vi "Agilent_33220A_FuncGen_TCP.vi"() -> ()   [LabVIEW 2019, in "Models of External Instruments.lvlib"]
uses:
  Models of External Instruments.lvlib
panel:
  out "remote address":string
  out "remote port":u16
  out "data out 2":string
  in  "data in":string
  out "bytes written":i32
  out "data out":string
  # "Output Configuration Commands\n\nOUTP ON\nOUTP OFF \n\nOUTP? --> 1 ON, 0 OFF\n\nOUTP:LOAD? -->yük empedansı\nOUTP:LOAD?  MAX--> maks yük empedansı\nOUTP:LOAD?  MIN--> min yük empedansı\n\nOUTP:POL? --> Normal or Inverted\nOUTP:POL INV -->Inverted waveform\nOUTP:POL?\n\nOUTP:POL NORM-->Normal Waveform\nOUTP:POL?\n\nOUTP:SYNC ON  -->Sync konnectörünü aktif eder\nOUTP:SYNC OFF -->Sync konnectörünü deaktif eder\nOUTP:SYNC? --> Sync konnectörünün durumu 1-ON, 0-OFF\n\nVOLT:UNIT? --> Voltaj biriminin durumu\nVOLT:UNIT VRMS -->birim Vrms\nVOLT:UNIT VPP -->birim Vpp\nVOLT:UNIT DBM -->birim dBm"
  # "Pulse Configuration Commands\n\nPULS:PER 5  --> saniye cinsinden darbe periydunun ayarı\nPULS:PER MIN --> Minimumu 200ns olarak ayarlar\nPULS:PER MAX --> Maxı 2000s olarak ayarlar\nPULS:PER? -*->pulse periyot durumu\n\nFUNC:PULSE:HOLD WID --> pulse genişliği şeklinde ayarla\nFUNC:PULSE:HOLD DCYC --> pulse duty cycle şeklinde ayarla\nFUNC:PULSE:HOLD -->Pulse ayar durumu\n\nFUNC:PULS:WIDT 5-->Pulse genişliği saniye cinsinden ayarla\nFUNC:PULS:WIDT MAX --> Pulse genişliğini max 1999.99 s olarak ayarla\nFUNC:PULS:WIDT MIN --> Pulse genişliğini min 20ns olarak ayarla\nFUNC:PULS:WIDT? --> Pulse genişliğinin durumu\n\nFUNC:PULS:DCYC 50-->Pulse duty cycle'ını oran cinsinden ayarla\nFUNC:PULS:DCYC MAX -->Pulse duty cycle'ını max 100% olarak ayarla\nFUNC:PULS:DCYC MIN --> Pulse duty cycle'ını  min 0% olarak ayarla\nFUNC:PULS:DCYC? -->  Pulse duty cycle'ının durumu\n\nFUNC:PULS:TRAN 50 --> düşen ve yükselen kenar için edge time'ı oran olarak ayarla\n                                             edge time from 5 ns to 100 ns\nFUNC:PULS:TRAN MAX --> edge time 100ns\nFUNC:PULS:TRAN MIN --> edge time 5ns\nFUNC:PULS:TRAN? -->edge time durumu"
  # "APPLy Command\n\nAPPL:SIN 5 KHZ, 3.0 VPP, -2.5 V\nAPPL?\n\nAPPL:SIN 5.0E+3, 3.0 VRMS, -2.5\nAPPL?\n\nAPPL:SQU 5.0E+3, 3.0, -2.5\nAPPL?"
  # "APPLy\n:SINusoid [<frequency> [,<amplitude> [,<offset>] ]]\n:SQUare [<frequency> [,<amplitude> [,<offset>] ]]\n:RAMP [<frequency> [,<amplitude> [,<offset>] ]]\n:PULSe [<frequency> [,<amplitude> [,<offset>] ]]\n:NOISe [<frequency|DEF>1 [,<amplitude> [,<offset>] ]]\n:DC [<frequency|DEF>1 [,<amplitude>|DEF>1 [,<offset>] ]]\n:USER [<frequency> [,<amplitude> [,<offset>] ]]\nAPPLy?"
  # "Low-Level Commands\n\nFUNC SIN --> Select sine wave function\nFREQ 5000 -->Set frequency to 5 kHz\nVOLT 3.0 --> Set amplitude to 3 Vpp\nVOLT:OFFS -2.5 --> Set offset to -2.5 Vdc\nAPPL?"
  # "*IDN? --> cihaz bilgileri: Agilent Technologies,33220A,<serial number>,f.ff-b.bb-aa-p\n                                            f.ff = Firmware revision number\n                                            b.bb = Boot kernel revision number\n                                            aa = ASIC revision number\n                                            p = Printed circuit board revision number\nSYSTem:VERSion? --> sistem verisyonu\n\nSYST:ERR? --> Hataları oku\n\nDISP ON--> ekranı aç\nDISP OFF--> ekranı kapat\nDISP? --> ekran durumu"
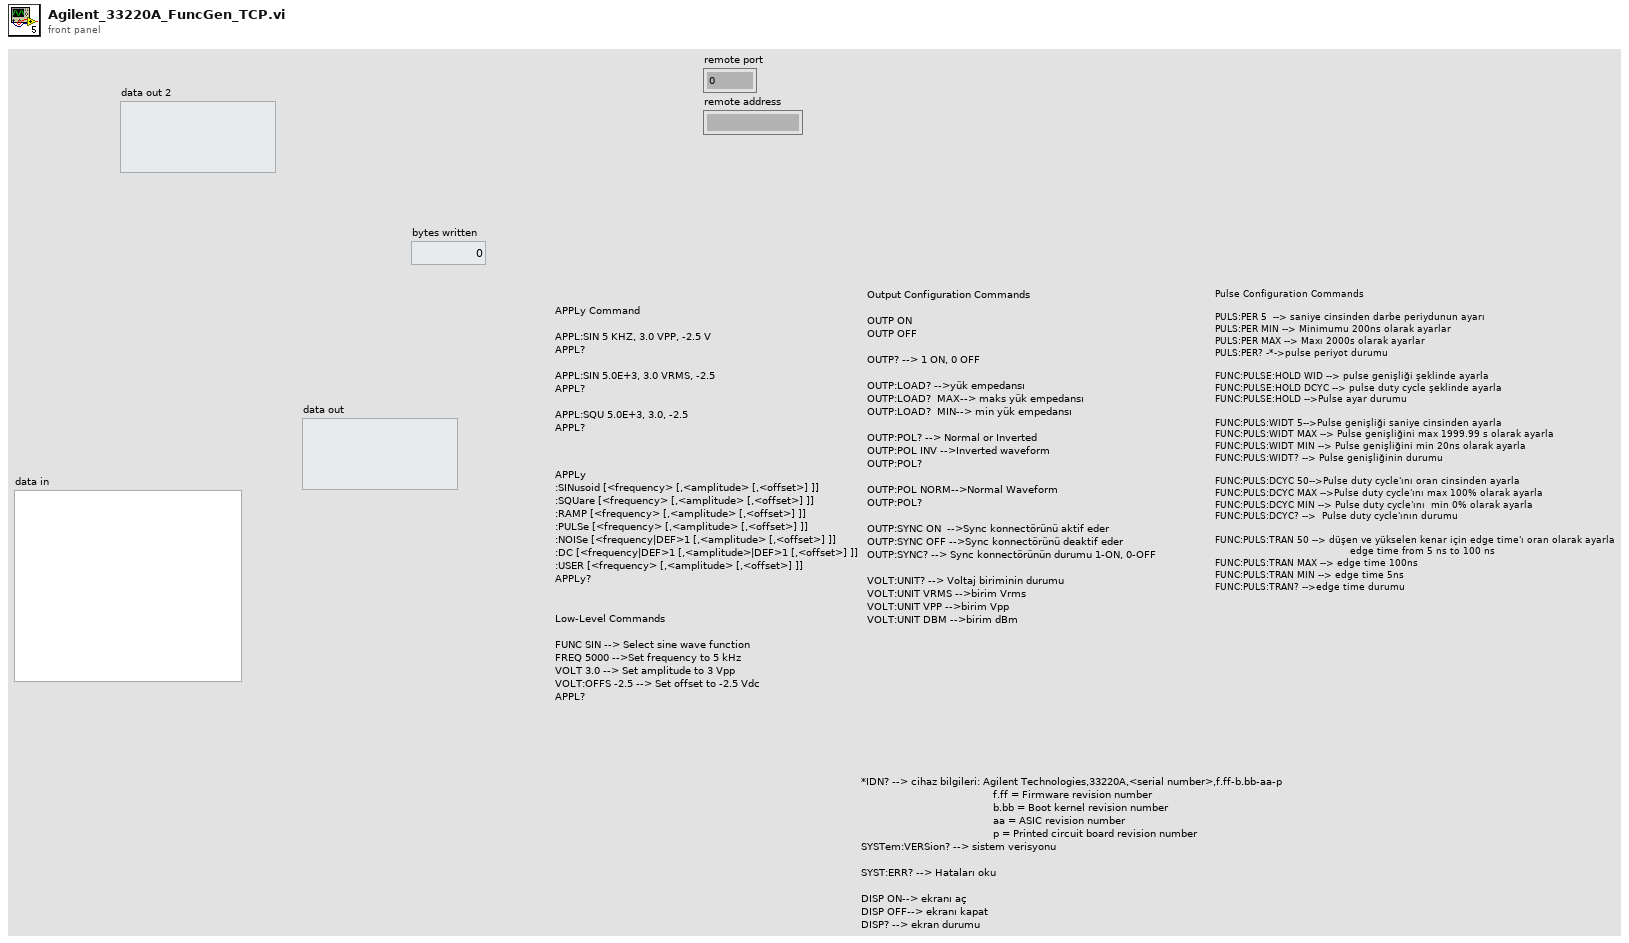
[diagram p1: front panel]
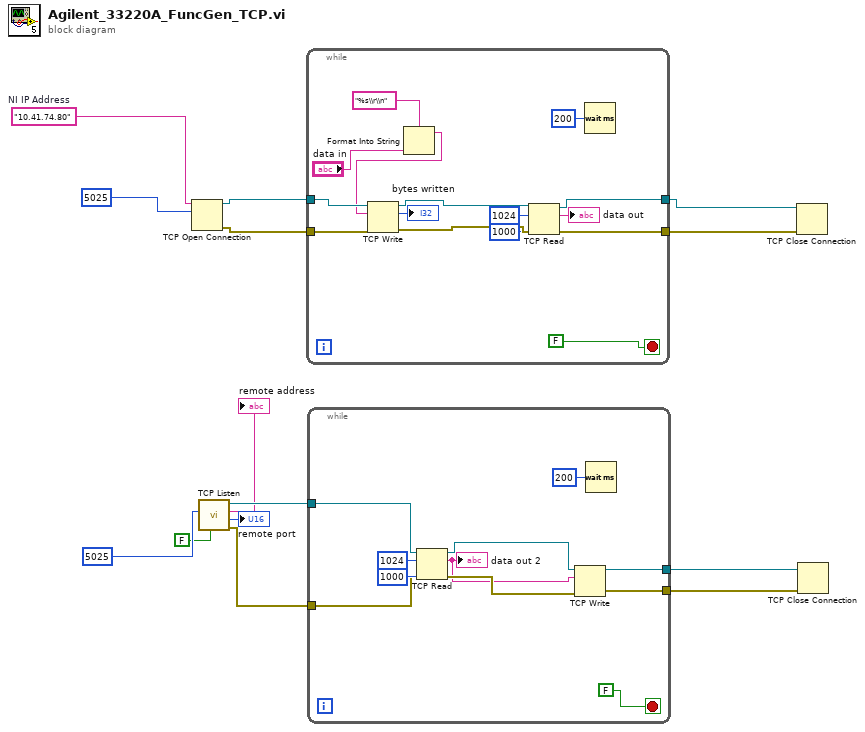
[diagram p0: block diagram]
diagram:
  w12 = "10.41.74.80"  # NI IP Address
  n1 = TCP Open Connection(address=w12, remote port or service name=u16 5025 ("port or service name")) -> (connection ID=w14:refnum<k5>, error out=w11:errorcluster)  [unwired: 3 in]
  n2 = call <vilib>:"TCP Listen.vi"("resolve remote address (T)"=FALSE, "port"=u16 5025 ("port or service name")) -> ("error out"=w7:errorcluster, "remote port"=→"remote port":u16, "remote address"=→"remote address":string, "connection ID"=w8:refnum<k5>)  [unwired: 5 in, 1 out]
  n3 = while {
    tunnel: w11 -> [w24]
    tunnel: [w16] -> w10
    tunnel: w14 -> [w29]
    tunnel: [w22] -> w9
    stop <- FALSE ("status") stop-if-true
    n4 = Format Into String(format string="%s\\r\\n", "data in") -> (resulting string=w25:string)  [unwired: 2 in, 1 out]
    n5 = TCP Write(connection ID=w29, data in=w25, error in (no error)=w24) -> (connection ID out=w20:refnum<k5>, bytes written=→"bytes written":i32, error out=w21:errorcluster)  [unwired: 1 in]
    n6 = TCP Read(connection ID=w20, bytes to read=1024, error in (no error)=w21, 9:1000 ("timeout ms (25000)")) -> (connection ID out=w22:refnum<k5>, data out=→"data out":string, error out=w16:errorcluster)  [unwired: 1 in]
    n7 = Wait (ms)(milliseconds to wait=u32 200) -> ()  [unwired: 1 out]
  }
  n8 = while {
    tunnel: w8 -> [w34]
    tunnel: w7 -> [w33]
    tunnel: [w32] -> w2
    tunnel: [w31] -> w1
    stop <- FALSE stop-if-true
    n9 = TCP Read(connection ID=w34, bytes to read=1024, error in (no error)=w33, 9:1000 ("timeout ms (25000)")) -> (connection ID out=w36:refnum<k5>, data out=w30:string, error out=w35:errorcluster)  [unwired: 1 in]
    "data out 2" <- w30
    n10 = TCP Write(connection ID=w36, data in=w30, error in (no error)=w35) -> (connection ID out=w32:refnum<k5>, error out=w31:errorcluster)  [unwired: 1 in, 1 out]
    n11 = Wait (ms)(milliseconds to wait=u32 200) -> ()  [unwired: 1 out]
  }
  n12 = TCP Close Connection(connection ID=w9, error in (no error)=w10) -> ()  [unwired: 1 in, 2 out]
  n13 = TCP Close Connection(connection ID=w2, error in (no error)=w1) -> ()  [unwired: 1 in, 2 out]
